vi "Inspect Stamp Fiducials.vi"(5 "Dispose Images?":bool, 6 "WorkTable Class in":refnum<class "WorkTable Class.lvclass">, 7 "Glue Pathways":T7 {"BBM Slot" items=["Slot 1", "Slot 2", "Slot 3", "Slot 4"]; "Weight Slot" items=["Slot 1", "Slot 2", "Slot 3", "Slot 4"]; "Glue Slot" items=["Slot 1", "Slot 2", "Slot 3", "Slot 4"]; "Stamp Slot" items=["Slot 1", "Slot 2", "Slot 3", "Slot 4"]; "HDI Slot" items=["Slot 1", "Slot 2", "Slot 3", "Slot 4"]}, 8 "error in":errorcluster, 9 "Console Log in":refnum<class "Console Log.lvclass">, 10 "Single Path in":T6, 11 "CameraTool in":refnum<class "CameraTool Class.lvclass">) -> (0 "error out":errorcluster, 1 "Console Log out":refnum<class "Console Log.lvclass">, 2 "Single Path out":T6, 3 "CameraTool out":refnum<class "CameraTool Class.lvclass">)   [LabVIEW 2011, in "Gluing Procedure.lvclass"]
uses:
  Gluing Procedure.lvclass
  UI typedefs/Glue Path.ctl
  Shared Components/WorkTable Class/WorkTable Class.lvclass
  Shared Components/CameraTool Class/CameraTool Class.lvclass
  Shared Components/Utils/Type Definitions/Part Fiducials.ctl
  Shared Components/Utils/Type Definitions/Fiducial Image.ctl
  Shared Components/Vec3d Class/Vec3d Class.lvclass
  Shared Components/Utils/Type Definitions/Physical Image.ctl
  <vilib>/vision/Image Controls.llb/IMAQ Image.ctl
  Shared Components/Utils/Type Definitions/Fiducial with Source.ctl
  Application Utilities/Console Log/Console Log.lvclass
  Shared Components/Config Manager Class/Type Definitions/Named Position.ctl
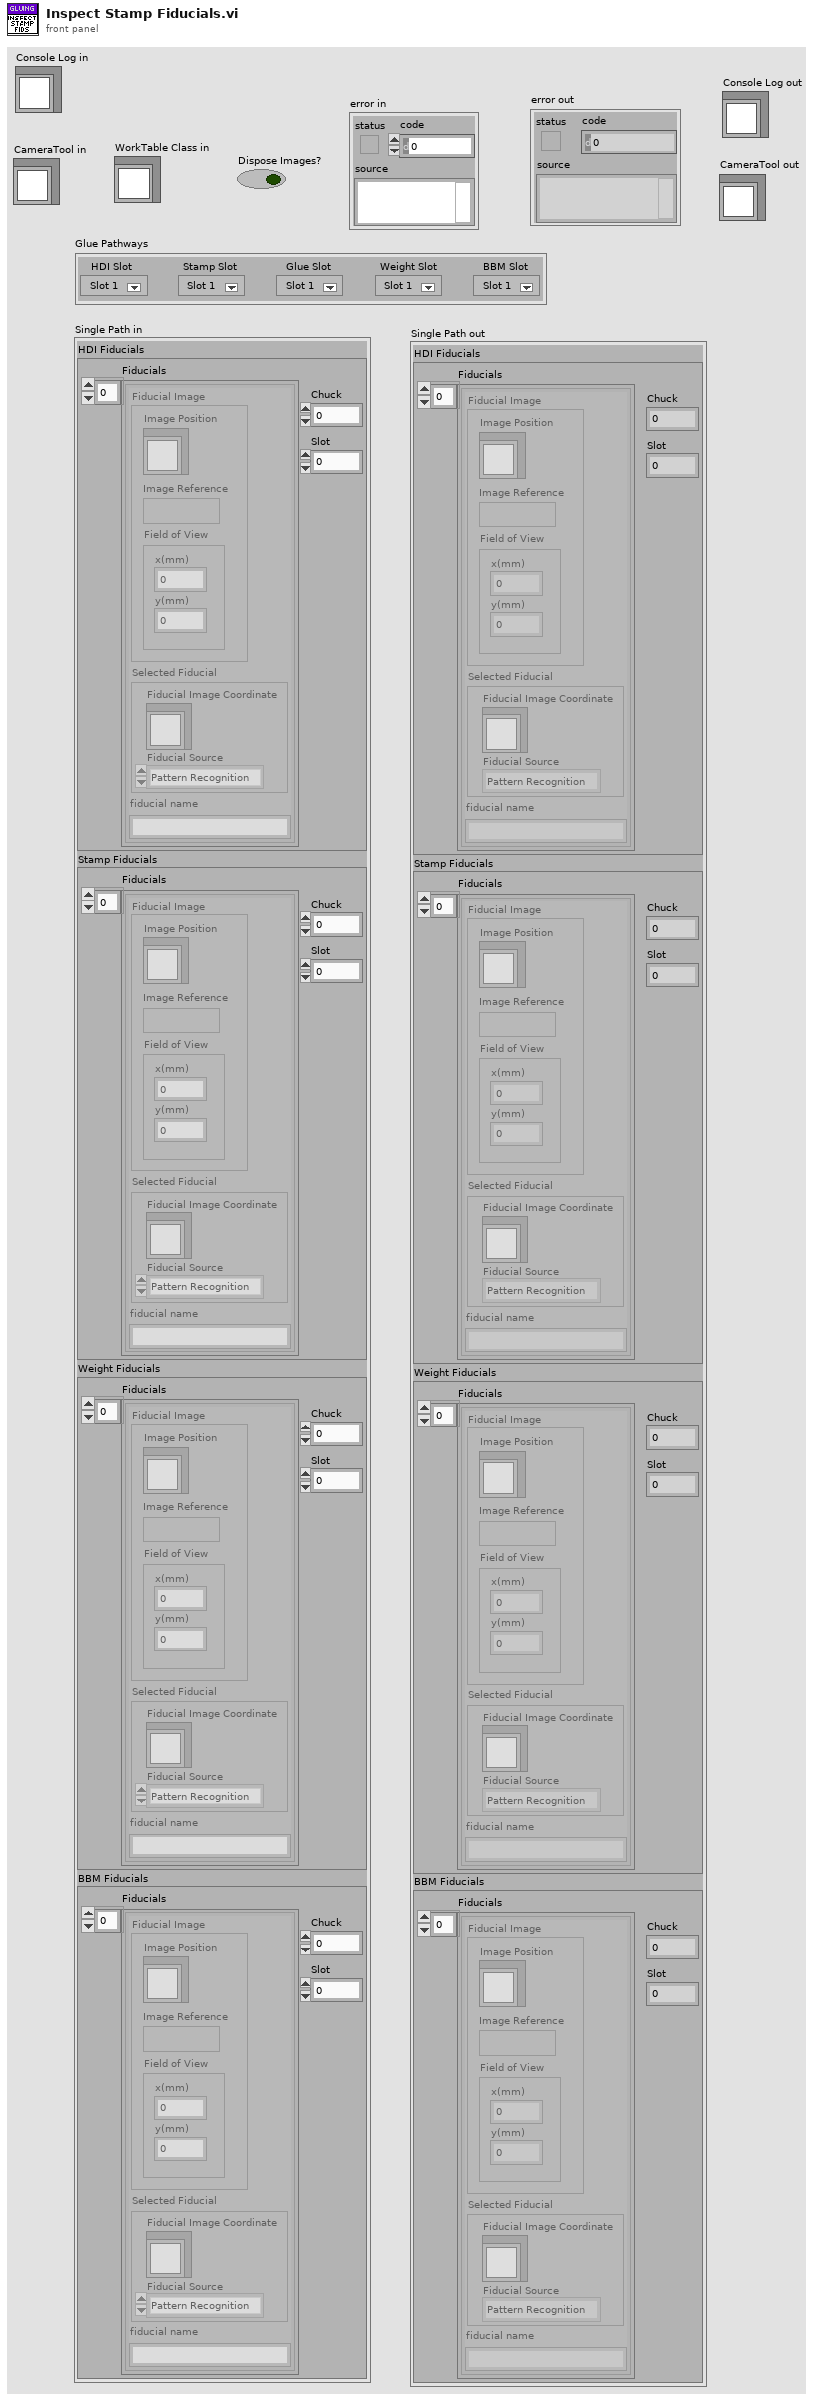
[diagram p1: front panel]
types:
  T1 = typedef "Part Fiducials.ctl" = cluster{"Fiducials":T2[], "Chuck":i32, "Slot":i32}
  T2 = typedef "Fiducial Image.ctl" = cluster{"Fiducial Image":T3, "Selected Fiducial":T5, "fiducial name":string}
  T3 = typedef "Physical Image.ctl" = cluster{"Image Position":refnum<class "Vec3d Class.lvclass">, "Image Reference":T4, "Field of View":cluster{"x(mm)":dbl, "y(mm)":dbl}}
  T4 = typedef "IMAQ Image.ctl" = refnum<image>
  T5 = typedef "Fiducial with Source.ctl" = cluster{"Fiducial Image Coordinate":refnum<class "Vec3d Class.lvclass">, "Fiducial Source":enum16{"Pattern Recognition", "User", "Error", "Default"}}
  T6 = cluster{"HDI Fiducials":T1, "Stamp Fiducials":T1, "Weight Fiducials":T1, "BBM Fiducials":T1}
  T7 = typedef "Glue Path.ctl" = cluster{"HDI Slot ":i32, "Stamp Slot":i32, "Glue Slot":i32, "Weight Slot":i32, "BBM Slot":i32}
  T8 = typedef "Named Position.ctl" = enum16{"home", "module_chuck_0", "module_chuck_1", "module_chuck_2", "module_chuck_3", "module_chuck_4", "glue_reservoir_chuck", "stamp_tool_chuck", "weight_tool_chuck", "needle_calibration", "tool_rack_pos_0_in", "tool_rack_pos_0_out", "tool_rack_pos_1_in", "tool_rack_pos_1_out", "tool_rack_pos_2_in", "tool_rack_pos_2_out", "front_load_position", "grabber_start_pos", "between_chuck_0_and_1", "between_chuck_2_and_3"}
  T9 = typedef "Worktable_Stamp.ctl" = cluster{"Stamp State":enum16{"Empty", "Populated", "Used"}, "Location/Orientation":T10, "Stamp Type":T11}
  T10 = typedef "Position_Orientation.ctl" = cluster{"Center":refnum<class "Vec3d Class.lvclass">, "Orientation":refnum<class "Orient3d Class.lvclass">}
  T11 = typedef "Stamp Type.ctl" = enum16{"Stamp 1", "Stamp 2", "Stamp 3", "Stamp 4", "Stamp 5"}
  T12 = typedef "Part Type.ctl" = enum16{"BBM", "HDI", "BARE HDI", "GLUERESERVOIR", "STAMP_1", "STAMP_2", "STAMP_3", "STAMP_4", "STAMP_5", "WEIGHT_1", "WEIGHT_2", "WEIGHT_3", "WEIGHT_4", "WEIGHT_5", "WEIGHT_6", "WEIGHT_7", "WEIGHT_8", "PICKER_TOOL", "GRABER_TOOL"}
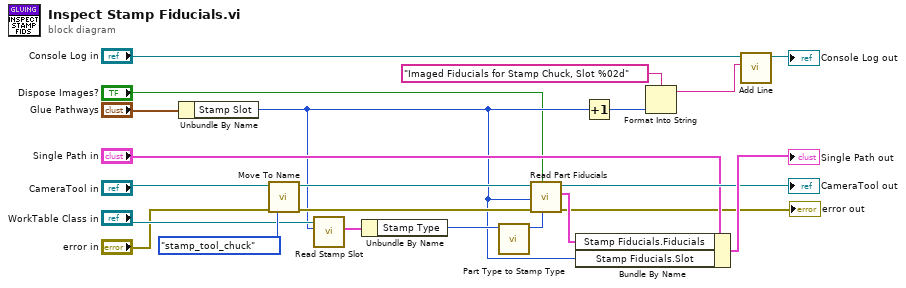
[diagram p0: block diagram]
diagram:
  n1 = Unbundle By Name("Glue Pathways") -> ("Stamp Slot"=w6:i32)
  n2 = call-dynamic "Move To Name.vi"("error in"="error in", "Destination"=Named_Position."stamp_tool_chuck", "Gantry in"="CameraTool in") -> ("error out"=w9:errorcluster, "Gantry out"=w13:refnum<class "CameraTool Class.lvclass">)  [unwired: 7 in]
  n3 = call "Read Stamp Slot.vi"("Stamp Slot"=w6, "WorkTable Class in"="WorkTable Class in") -> ("Stamp Slot"=w21:T9)  [unwired: 7 in, 2 out]
  n4 = Unbundle By Name(w21) -> ("Stamp Type"=w20:T11)
  n5 = call "Part Type to Stamp Type.vi"("Stamp Type"=w20) -> ("Part Type"=w19:T12)  [unwired: 9 in, 1 out]
  n6 = call-dynamic "Read Part Fiducials.vi"("Part Type"=w19, "Dispose Images?"="Dispose Images?", "error in"=w9, "Slot"=w6, "CameraTool in"=w13) -> ("error out"=→"error out":errorcluster, "Fiducials"=w18:T2[], "CameraTool out"=→"CameraTool out":refnum<class "CameraTool Class.lvclass">)  [unwired: 4 in]
  n7 = Bundle By Name(cluster="Single Path in", "Stamp Fiducials.Fiducials"=w18, "Stamp Fiducials.Slot"=w6) -> (→"Single Path out":T6)
  n8 = Increment(x=w6) -> (x+1=w5:i32)
  n9 = Format Into String(format string="Imaged Fiducials for Stamp Chuck, Slot %02d", w5) -> (resulting string=w3:string)  [unwired: 2 in, 1 out]
  n10 = call "Add Line.vi"("String"=w3, "Console Log in"="Console Log in") -> ("Console Log out"=→"Console Log out":refnum<class "Console Log.lvclass">)  [unwired: 8 in, 1 out]
